vi "Recipe Label Changed.vi"(8 "error in (no error)":errorcluster, 9 "New Label":string, 10 "Old Label":string, 11 "Main Window Interface in":refnum<class "Main Window Interface.lvclass">) -> (0 "error out":errorcluster, 3 "Main Window Interface out":refnum<class "Main Window Interface.lvclass">)   [LabVIEW 2021, in "Recipe.lvlib" / "Main Window Interface.lvclass"]
uses:
  Main Window Interface.lvclass
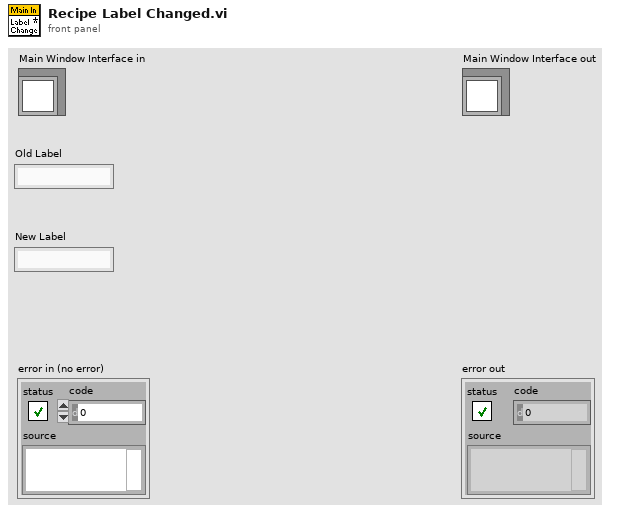
[diagram p1: front panel]
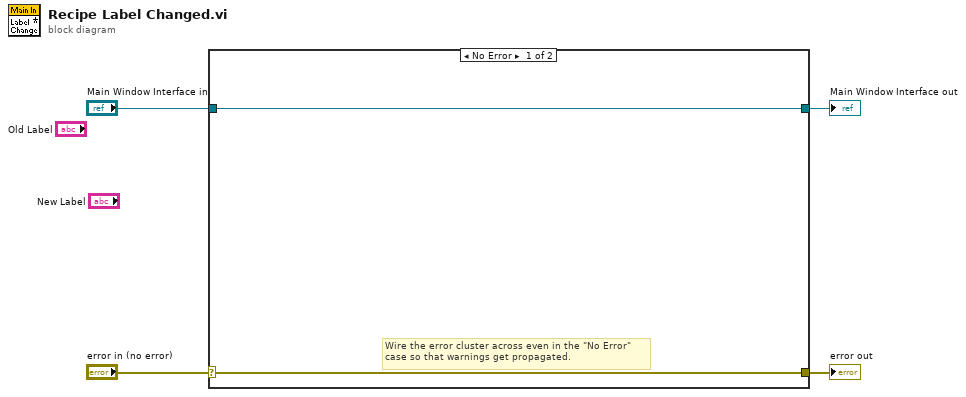
[diagram p0: block diagram]
diagram:
  n1 = case shown="No Error" "error in (no error)" {
    selector: "error in (no error)" -> [w5 w8]
    tunnel: [w5 w8] -> w3
    tunnel: [w6 w7] -> w1
    tunnel: "Main Window Interface in" -> [w6 w7]
    frame No Error {
      # "Wire the error cluster across even in the \"No Error\"\ncase so that warnings get propagated."
    }
    frame Error {
    }
  }
  "error out" <- w3
  "Main Window Interface out" <- w1
